vi "ASI Get Data After Exp.vi"(9 "lBuffSize":i32, 11 "iCameraID":i32) -> (1 "pBuffer out":u8[](array[numeric]), 3 "function return":i32)   [LabVIEW 2023, in "ASICamera2_no_err.lvlib"]
doc: "ASICAMERA_API ASI_ERROR_CODE ASIGetDataAfterExp(int iCameraID, unsigned char* pBuffer, long lBuffSize);"
uses:
  ASICamera2_no_err.lvlib
  LabviewDAQ-master/ConcreteClasses/ConcreteInstrumentClasses/CameraClasses/ZWO_ASI_LV/Labview_ASI_demo_64bit_221128/user.lib/ASICamera2_no_err/ASICamera2.dll
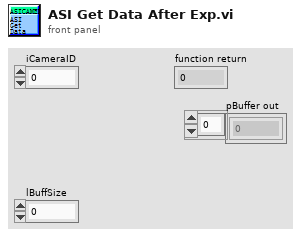
[diagram p1: front panel]
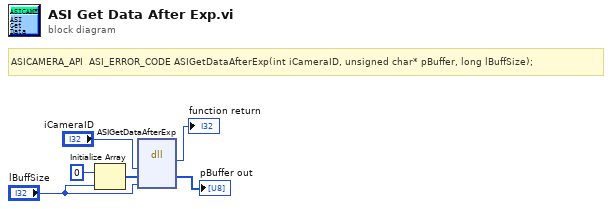
[diagram p0: block diagram]
diagram:
  # "ASICAMERA_API  ASI_ERROR_CODE ASIGetDataAfterExp(int iCameraID, unsigned char* pBuffer, long lBuffSize);"
  n1 = Initialize Array(u8 0, "lBuffSize") -> (w2:u8[])
  n2 = dll-call lib="W:/Quant_Opt_Group/Group/Alex/LabviewDAQ-master/ConcreteClasses/ConcreteInstrumentClasses/CameraClasses/ZWO_ASI_LV/Labview_ASI_demo_64bit_221128/user.lib/ASICamera2_no_err/ASICamera2.*" fn="ASIGetDataAfterExp"("iCameraID"="iCameraID", "pBuffer"=w2, "lBuffSize"="lBuffSize") -> ("返回类型"=→"function return":i32, "pBuffer"=→"pBuffer out":u8[])  [unwired: 5 in, 2 out]
